vi "read error log.vi"() -> ()   [LabVIEW 2018]
panel:
  out "subarray 3":string[](array[string])
  out "subarray 2":string[](array[string])
  out "subarray":string[](array[string])
  out "Location Cluster out":T1
  in  "Tab Control":enum32{"Page 1", "Page 2", "Page 3"}(tab)
  out "Display":string[][](table)
  out "raw screen":string
  out "read":string
  out "text 2":string
  out "text":string
  out "all rows":string[][](array[string])
  out "Selection Position":cluster{i32, i32}={6, 2}
  in  "Stop":bool
  out "error out":errorcluster
  out "Source":string
  out "Code":string
  out "Timestamp":string
  in  "Numeric":i32
  # "is screen dimension check not working?? number of columns are counted in update display..."
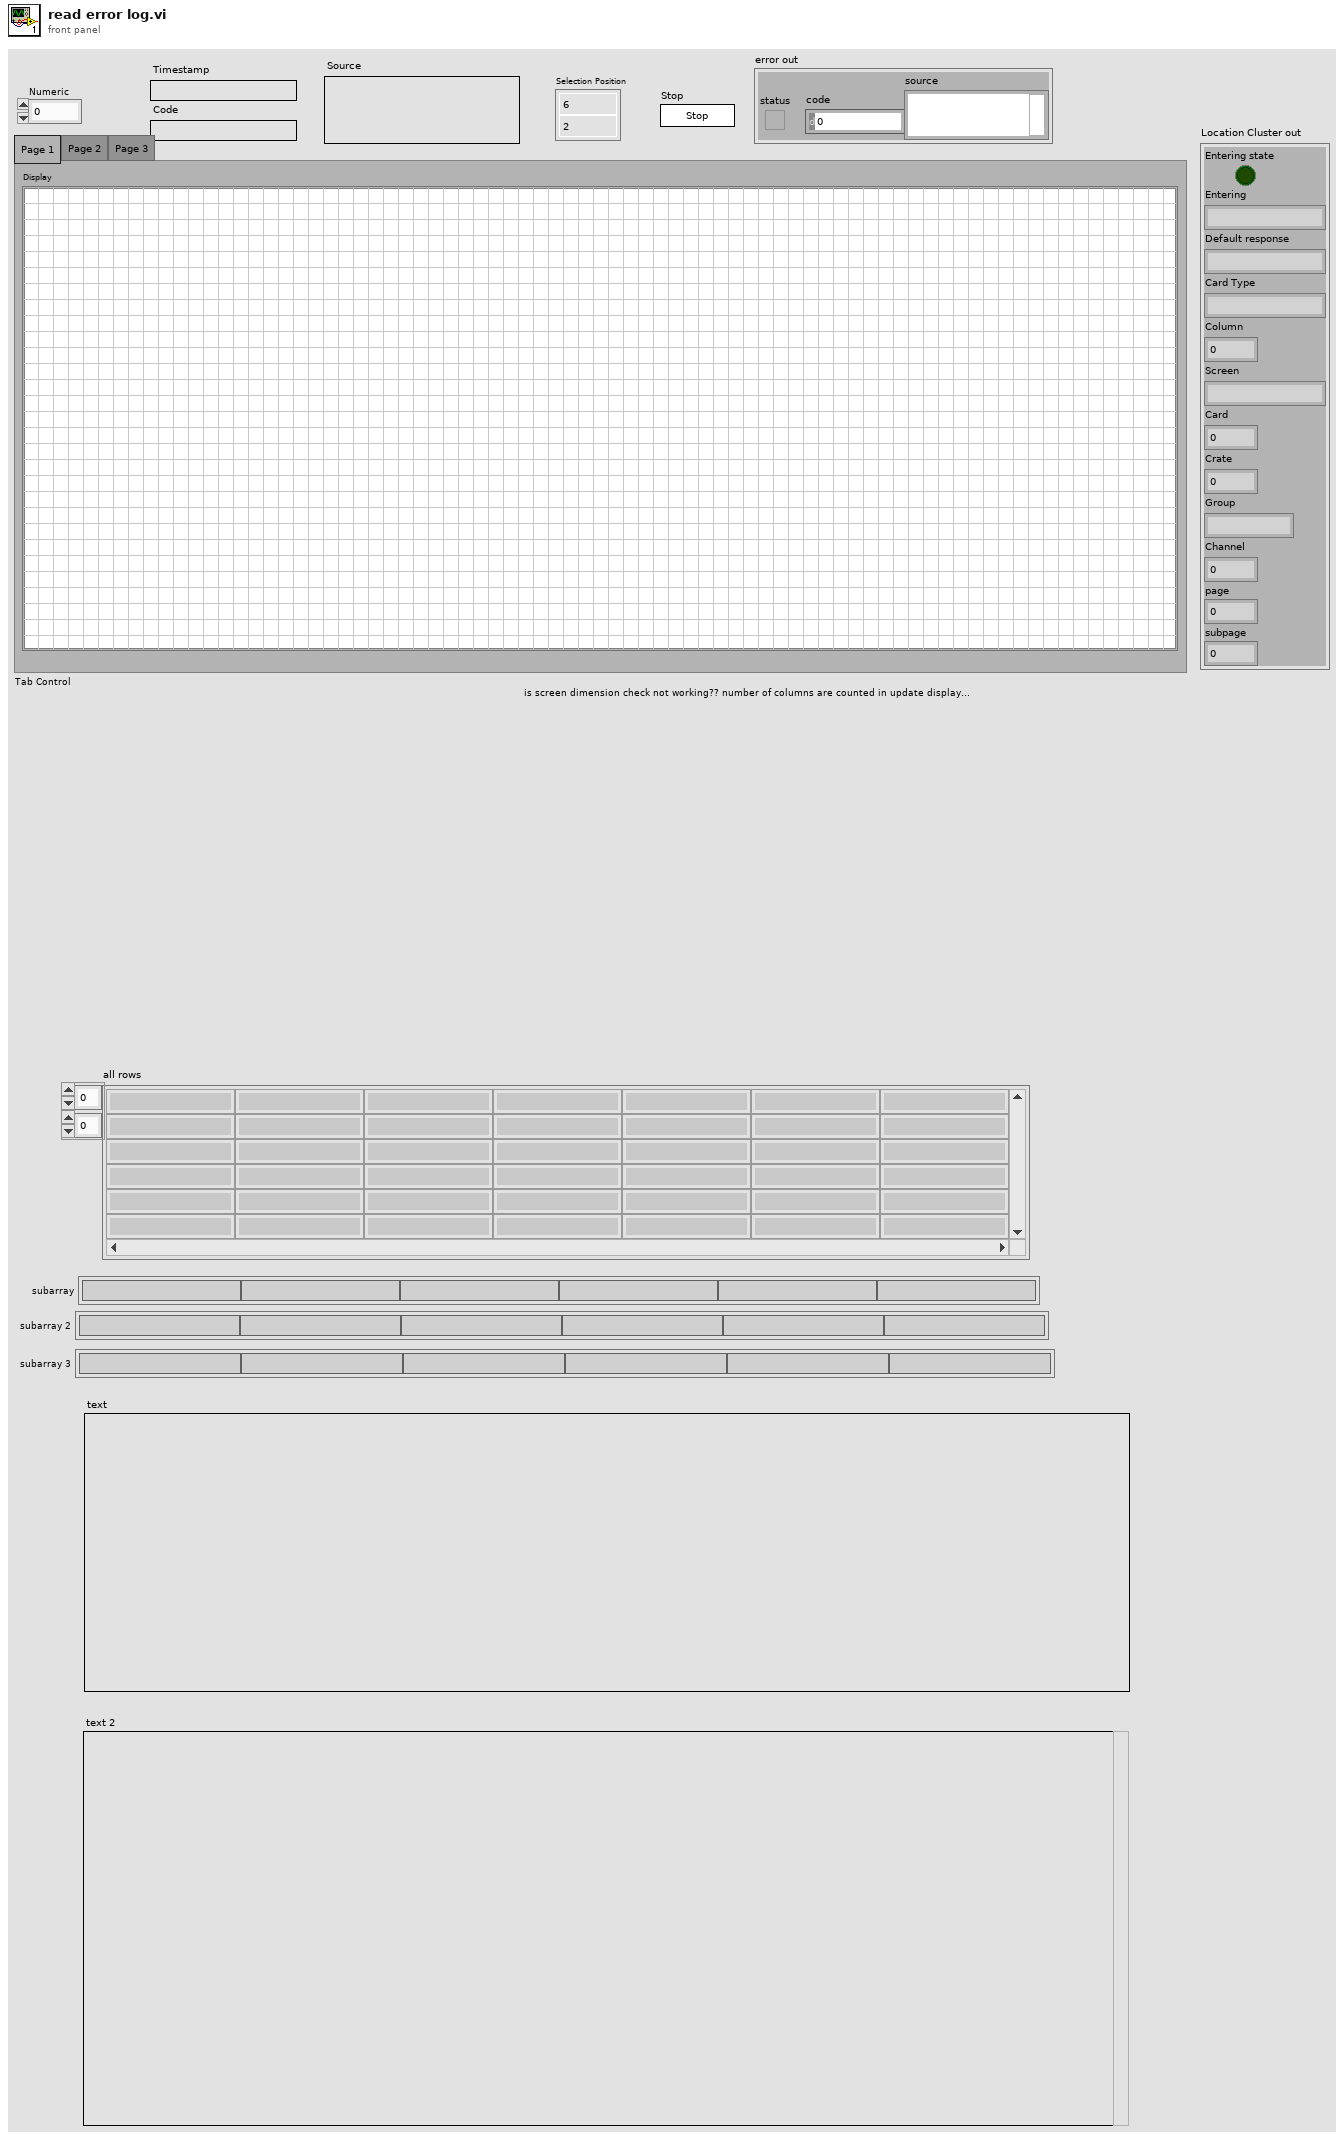
[diagram p1: front panel]
types:
  T1 = cluster{"Screen":string, "Crate":i32, "page":i32, "subpage":i32, "Entering state":bool, "Entering":string, "Default response":string, "Card":i32, "Channel":i32, "Card Type":string, "Column":i32, "Group":string}
  T2 = typedef "location cluster.ctl" = cluster{"Column":i32, "Card Type":string, "Channel":i32, "Card":i32, "Default response":string, "Entering":string, "Entering state":bool, "subpage":i32, "page":i32, "Crate":i32, "Screen":string, "Group":string, "Global HV Enable":bool}
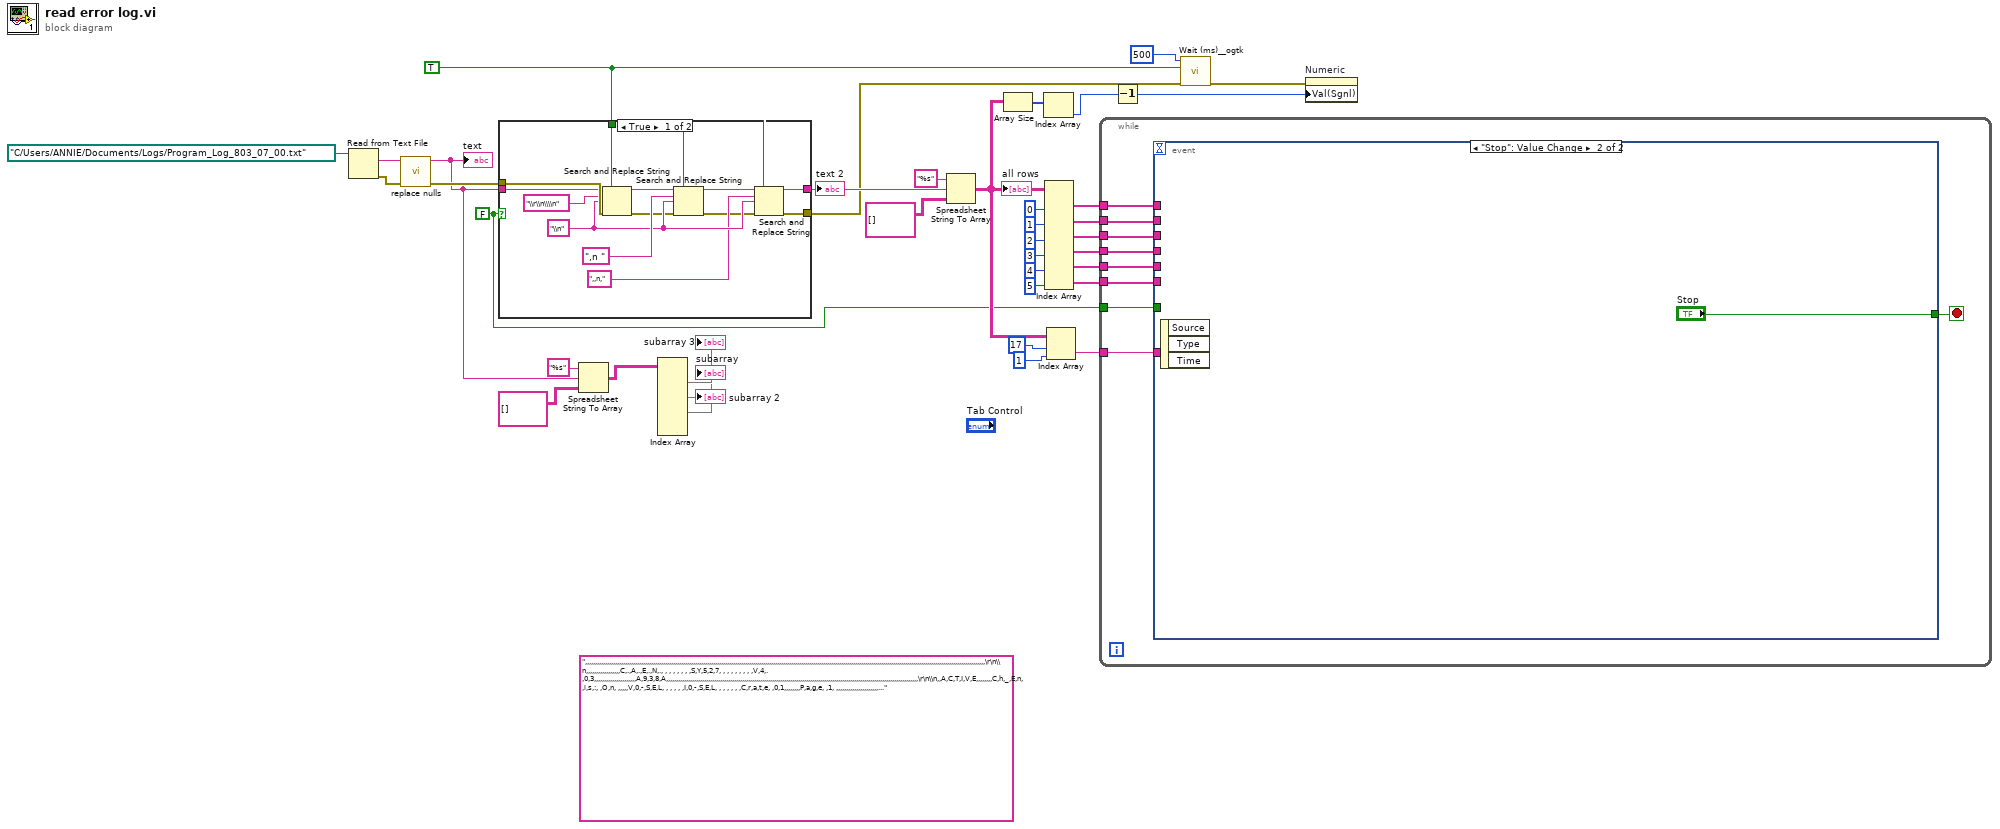
[diagram p0: block diagram]
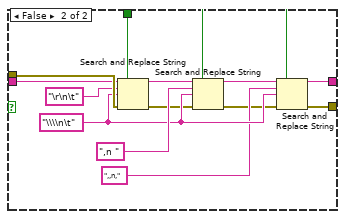
[diagram p2: hidden frame]
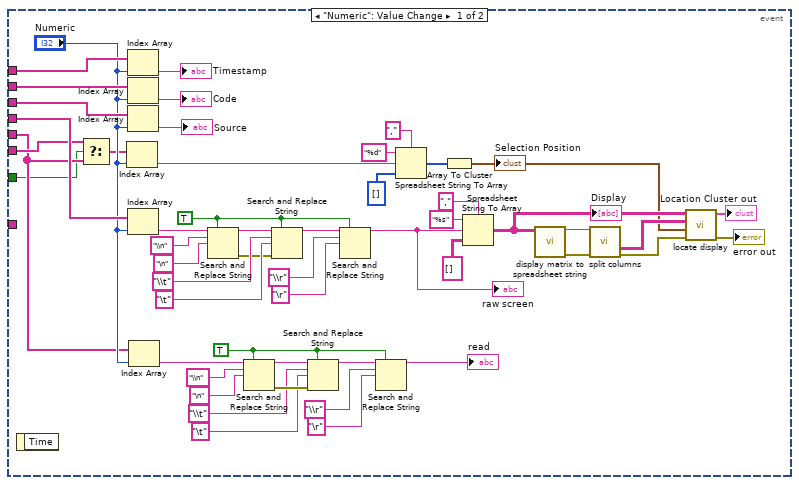
[diagram p3: hidden frame]
diagram:
  w1 = FALSE
  w17 = TRUE ("replace all? (F)")
  (unwired) ",,,,,,,,,,,,,,,,,,,,,,,,,,,,,,,,,,,,,,,,,,,,,,,,,,,,,,,,,,,,,,,,,,,,,,,,,,,,,,,,,,,,,,,,,,,,,,,,,,,,,,,,,,,,,,,,,,,,,,,,,,,,,,,,,,,,,,,,,,,,,,,,,,,,,,,,,,,,,,,,,,,,,,,,,,,,,,,,,,,,,,,,,,,,,,,,,,,,,,,,\r\n\\n,,,,,,,,,,,,,,,,,C,.,A,.,E,.,N,., , , , , , , ,S,Y,5,2,7, , , , , , , , ,V,4,.,0,3,,,,,,,,,,,,,,,,,,,,,A,9,3,8,A,,,,,,,,,,,,,,,,,,,,,,,,,,,,,,,,,,,,,,,,,,,,,,,,,,,,,,,,,,,,,,,,,,,,,,,,,,,,,,,,,,,,,,,,,,,,,,,,,,,,,,,,,,,,,,,,,,,,,,,,,,,,,,\r\n\\n,,A,C,T,I,V,E,,,,,,,,C,h,_,E,n, ,i,s,:, ,O,n, ,,,,,V,0,-,S,E,L, , , , , ,I,0,-,S,E,L, , , , , , ,C,r,a,t,e, ,0,1,,,,,,,,P,a,g,e, ,1, ,,,,,,,,,,,,,,,,,,,,,,,,,,,,,,,,,,,,,,,,,,,,,,,,,,,,,,,,,,,,,,,,,,,,,,,,,,,,,,,,,,,,,,,,,,,,,,,,,,,,,,,,,,,,,,,,,,,,,,,,,,,,\r\n\\n,,,,,,,,,,,,,,,,,,,,,,,,,,,,,,,,,,,,,,,,,,,,,,,,,,,,,,,,,,,,,,,,,,,,,,,,,,,,,,,,,,,,,,,,,,,,,,,,,,,,,,,,,,,,,,,,,,,,,,,,,,,,,,,,,,,,,,,,,,,,,,,,,,,,,,,,,,,,,,,,,,,,,,,,,,,,,,,,,,,,,,,,,,,,,,,,,,,,,,,,\r\n\\n, ,C,h,a,n,n,e,l, , , , , ,S,V,m,a,x, , ,R,u,p, , ,R,d,w,n, , ,T,r,i,p, ,T,r,i,p,E,x, ,P,r,O,n, ,P,r,O,f,f, ,P,o,n, , ,P,d,w,n, ,P,s,w,d, ,O,n,/,O,f,f, , ,C,h,#,,,,,,,,,,,,,,,,,,,,,,,,,,,,,,,,,,,,,,,,,,,,,,,,,,,,,,,,,,,,,,,,,,,,,,,,,,,,,,,,,,,,,,,,,,,,,,,,,,,,,,,,,,,,,,,,,,,,,,,,\r\n\\n, ,C,H,A,N,N,E,L,1,6, , , , ,2,0,0,0, , ,1,0,0, , ,1,0,0, , ,0,1,0,.,0, , , ,-,-, , , , ,0,1, , , ,0,1, , , ,O,f,f, , ,R,d,w,n, , , , , , , , , , , , , ,1,.,1,6,,,,,,,,,,,,,,,,,,,,,,,,,,,,,,,,,,,,,,,,,,,,,,,,,,,,,,,,,,,,,,,,,,,,,,,,,,,,,,,,,,,,,,,,,,,,,,,,,,,,,,,,,,,,,,,,,,,,,,,,\r\n\\n, ,C,H,A,N,N,E,L,1,7, , , , ,2,0,0,0, , ,1,0,0, , ,1,0,0, , ,0,1,0,.,0, , , ,-,-, , , , ,0,1, , , ,0,1, , , ,O,f,f, , ,R,d,w,n, , , , , , , , , , , , , ,1,.,1,7,,,,,,,,,,,,,,,,,,,,,,,,,,,,,,,,,,,,,,,,,,,,,,,,,,,,,,,,,,,,,,,,,,,,,,,,,,,,,,,,,,,,,,,,,,,,,,,,,,,,,,,,,,,,,,,,,,,,,,,,\r\n\\n, ,C,H,A,N,N,E,L,1,8, , , , ,2,0,0,0, , ,1,0,0, , ,1,0,0, , ,0,1,0,.,0, , , ,-,-, , , , ,0,1, , , ,0,1, , , ,O,f,f, , ,R,d,w,n, , , , , , , , , , , , , ,1,.,1,8,,,,,,,,,,,,,,,,,,,,,,,,,,,,,,,,,,,,,,,,,,,,,,,,,,,,,,,,,,,,,,,,,,,,,,,,,,,,,,,,,,,,,,,,,,,,,,,,,,,,,,,,,,,,,,,,,,,,,,,,\r\n\\n, ,C,H,A,N,N,E,L,1,9, , , , ,2,0,0,0, , ,1,0,0, , ,1,0,0, , ,0,1,0,.,0, , , ,-,-, , , , ,0,1, , , ,0,1, , , ,O,f,f, , ,R,d,w,n, , , , , , , , , , , , , ,1,.,1,9,,,,,,,,,,,,,,,,,,,,,,,,,,,,,,,,,,,,,,,,,,,,,,,,,,,,,,,,,,,,,,,,,,,,,,,,,,,,,,,,,,,,,,,,,,,,,,,,,,,,,,,,,,,,,,,,,,,,,,,,\r\n\\n, ,C,H,A,N,N,E,L,2,0, , , , ,2,0,0,0, , ,1,0,0, , ,1,0,0, , ,0,1,0,.,0, , , ,-,-, , , , ,0,1, , , ,0,1, , , ,O,f,f, , ,R,d,w,n, , , , , , , , , , , , , ,1,.,2,0,,,,,,,,,,,,,,,,,,,,,,,,,,,,,,,,,,,,,,,,,,,,,,,,,,,,,,,,,,,,,,,,,,,,,,,,,,,,,,,,,,,,,,,,,,,,,,,,,,,,,,,,,,,,,,,,,,,,,,,,\r\n\\n, ,C,H,A,N,N,E,L,2,1, , , , ,2,0,0,0, , ,1,0,0, , ,1,0,0, , ,0,1,0,.,0, , , ,-,-, , , , ,0,1, , , ,0,1, , , ,O,f,f, , ,R,d,w,n, , , , , , , , , , , , , ,1,.,2,1,,,,,,,,,,,,,,,,,,,,,,,,,,,,,,,,,,,,,,,,,,,,,,,,,,,,,,,,,,,,,,,,,,,,,,,,,,,,,,,,,,,,,,,,,,,,,,,,,,,,,,,,,,,,,,,,,,,,,,,,\r\n\\n, ,C,H,A,N,N,E,L,2,2, , , , ,2,0,0,0, , ,1,0,0, , ,1,0,0, , ,0,1,0,.,0, , , ,-,-, , , , ,0,1, , , ,0,1, , , ,O,f,f, , ,R,d,w,n, , , , , , , , , , , , , ,1,.,2,2,,,,,,,,,,,,,,,,,,,,,,,,,,,,,,,,,,,,,,,,,,,,,,,,,,,,,,,,,,,,,,,,,,,,,,,,,,,,,,,,,,,,,,,,,,,,,,,,,,,,,,,,,,,,,,,,,,,,,,,,\r\n\\n, ,C,H,A,N,N,E,L,2,3, , , , ,2,0,0,0, , ,1,0,0, , ,1,0,0, , ,0,1,0,.,0, , , ,-,-, , , , ,0,1, , , ,0,1, , , ,O,f,f, , ,R,d,w,n, , , , , , , , , , , , , ,1,.,2,3,,,,,,,,,,,,,,,,,,,,,,,,,,,,,,,,,,,,,,,,,,,,,,,,,,,,,,,,,,,,,,,,,,,,,,,,,,,,,,,,,,,,,,,,,,,,,,,,,,,,,,,,,,,,,,,,,,,,,,,,\r\n\\n, ,C,H,A,N,N,E,L,2,4, , , , ,2,0,0,0, , ,1,0,0, , ,1,0,0, , ,0,1,0,.,0, , , ,-,-, , , , ,0,1, , , ,0,1, , , ,O,f,f, , ,R,d,w,n, , , , , , , , , , , , , ,1,.,2,4,,,,,,,,,,,,,,,,,,,,,,,,,,,,,,,,,,,,,,,,,,,,,,,,,,,,,,,,,,,,,,,,,,,,,,,,,,,,,,,,,,,,,,,,,,,,,,,,,,,,,,,,,,,,,,,,,,,,,,,,\r\n\\n, ,C,H,A,N,N,E,L,0,0, , , , ,2,0,0,0, , ,1,0,0, , ,1,0,0, , ,0,1,0,.,0, , , ,-,-, , , , ,0,1, , , ,0,1, , , ,O,f,f, , ,R,d,w,n, , , , , , , , , , , , , ,2,.,0,0,,,,,,,,,,,,,,,,,,,,,,,,,,,,,,,,,,,,,,,,,,,,,,,,,,,,,,,,,,,,,,,,,,,,,,,,,,,,,,,,,,,,,,,,,,,,,,,,,,,,,,,,,,,,,,,,,,,,,,,,\r\n\\n, ,C,H,A,N,N,E,L,0,1, , , , ,2,0,0,0, , ,1,0,0, , ,1,0,0, , ,0,1,0,.,0, , , ,-,-, , , , ,0,1, , , ,0,1, , , ,O,f,f, , ,R,d,w,n, , , , , , , , , , , , , ,2,.,0,1,,,,,,,,,,,,,,,,,,,,,,,,,,,,,,,,,,,,,,,,,,,,,,,,,,,,,,,,,,,,,,,,,,,,,,,,,,,,,,,,,,,,,,,,,,,,,,,,,,,,,,,,,,,,,,,,,,,,,,,,\r\n\\n, ,C,H,A,N,N,E,L,0,2, , , , ,2,0,0,0, , ,1,0,0, , ,1,0,0, , ,0,1,0,.,0, , , ,-,-, , , , ,0,1, , , ,0,1, , , ,O,f,f, , ,R,d,w,n, , , , , , , , , , , , , ,2,.,0,2,,,,,,,,,,,,,,,,,,,,,,,,,,,,,,,,,,,,,,,,,,,,,,,,,,,,,,,,,,,,,,,,,,,,,,,,,,,,,,,,,,,,,,,,,,,,,,,,,,,,,,,,,,,,,,,,,,,,,,,,\r\n\\n, ,C,H,A,N,N,E,L,0,3, , , , ,2,0,0,0, , ,1,0,0, , ,1,0,0, , ,0,1,0,.,0, , , ,-,-, , , , ,0,1, , , ,0,1, , , ,O,f,f, , ,R,d,w,n, , , , , , , , , , , , , ,2,.,0,3,,,,,,,,,,,,,,,,,,,,,,,,,,,,,,,,,,,,,,,,,,,,,,,,,,,,,,,,,,,,,,,,,,,,,,,,,,,,,,,,,,,,,,,,,,,,,,,,,,,,,,,,,,,,,,,,,,,,,,,,\r\n\\n, ,C,H,A,N,N,E,L,0,4, , , , ,2,0,0,0, , ,1,0,0, , ,1,0,0, , ,0,1,0,.,0, , , ,-,-, , , , ,0,1, , , ,0,1, , , ,O,f,f, , ,R,d,w,n, , , , , , , , , , , , , ,2,.,0,4,,,,,,,,,,,,,,,,,,,,,,,,,,,,,,,,,,,,,,,,,,,,,,,,,,,,,,,,,,,,,,,,,,,,,,,,,,,,,,,,,,,,,,,,,,,,,,,,,,,,,,,,,,,,,,,,,,,,,,,,\r\n\\n, ,C,H,A,N,N,E,L,0,5, , , , ,1,8,0,0, , ,1,0,0, , ,1,0,0, , ,0,1,0,.,0, , , ,-,-, , , , ,0,1, , , ,0,1, , , ,O,f,f, , ,R,d,w,n, , , , , , , , , , , , , ,2,.,0,5,,,,,,,,,,,,,,,,,,,,,,,,,,,,,,,,,,,,,,,,,,,,,,,,,,,,,,,,,,,,,,,,,,,,,,,,,,,,,,,,,,,,,,,,,,,,,,,,,,,,,,,,,,,,,,,,,,,,,,,,\r\n\\n, ,C,H,A,N,N,E,L,0,6, , , , ,1,8,0,0, , ,1,0,0, , ,1,0,0, , ,0,1,0,.,0, , , ,-,-, , , , ,0,1, , , ,0,1, , , ,O,f,f, , ,R,d,w,n, , , , , , , , , , , , , ,2,.,0,6,,,,,,,,,,,,,,,,,,,,,,,,,,,,,,,,,,,,,,,,,,,,,,,,,,,,,,,,,,,,,,,,,,,,,,,,,,,,,,,,,,,,,,,,,,,,,,,,,,,,,,,,,,,,,,,,,,,,,,,,\r\n\\n,,,,,,,,,,,,,,,,,,,,,,,,,,,,,,,,,,,,,,,,,,,,,,,,,,,,,,,,,,,,,,,,,,,,,,,,,,,,,,,,,,,,,,,,,,,,,,,,,,,,,,,,,,,,,,,,,,,,,,,,,,,,,,,,,,,,,,,,,,,,,,,,,,,,,,,,,,,,,,,,,,,,,,,,,,,,,,,,,,,,,,,,,,,,,,,,,,,,,,,,\r\n\\n,,,,,,,,,,,,,,,,,,,,,,,,,,,,,,,,,,,,,,,,,,,,,,,,,,,,,,,,,,,,,,,,,,,,,,,,,,,,,,,,,,,,,,,,,,,,,,,,,,,,,,,,,,,,,,,,,,,,,,,,,,,,,,,,,,,,,,,,,,,,,,,,,,,,,,,,,,,,,,,,,,,,,,,,,,,,,,,,,,,,,,,,,,,,,,,,,,,,,,,,\r\n\\n,,,,,,,,,,,,,,,,,,,,,,,,,,,,,,,,,,,,,,,,,,,,,,,,,,,,,,,,,,,,,,,,,,,,,,,,,,,,,,,,,,,,,,,,,,,,,,,,,,,,,,,,,,,,,,,,,,,,,,,,,,,,,,,,,,,,,,,,,,,,,,,,,,,,,,,,,,,,,,,,,,,,,,,,,,,,,,,,,,,,,,,,,,,,,,,,,,,,,,,,\r\n\\n, ,Q,u,i,t, ,E,d,i,t, ,C,h,a,n,g,e, ,A,d,d, ,I,n,s,e,r,t, ,R,e,p,l,a,c,e, ,D,e,l,e,t,e, ,U,p,d,a,t,e, ,N,e,x,t, ,P,r,e,v, ,M,o,r,e, ,S,w,i,t,c,h,,,,,,,,,,,,,,,,,,,,,,,,,,,,,,,,,,,,,,,,,,,,,,,,,,,,,,,,,,,,,,,,,,,,,,,,,,,,,,,,,,,,,,,,,,,,,,,,,,,,,,,,,,,,,,,,,,,,,,,,,,,,,,,,\r\n\\n,,,,,,,,,,,,,,,,,,,,,,,,,,,,,,,,,,,,,,,,,,,,,,,,,,,,,,,,,,,,,,,,,,,,,,,,,,,,,,,,,,,,,,,,,,,,,,,,,,,,,,,,,,,,,,,,,,,,,,,,,,,,,,,,,,,,,,,,,,,,,,,,,,,,,,,,,,,,,,,,,,,,,,,,,,,,,,,,,,,,,,,,,,,,,,,,,,,,,,,,\r\n\\n,,,,,,,,,,,,,,,,,,,,,,,,,,,,,,,,,,,,,,,,,,,,,,,,,,,,,,,,,,,,,,,,,,,,,,,,,,,,,,,,,,,,,,,,,,,,,,,,,,,,,,,,,,,,,,,,,,,,,,,,,,,,,,,,,,,,,,,,,,,,,,,,,,,,,,,,,,,,,,,,,,,,,,,,,,,,,,,,,,,,,,,,,,,,,,,,,,,,,,,,\r\n\\n,,,,,,,,,,,,,,,,,,,,,,,,,,,,,,,,,,,,,,,,,,,,,,,,,,,,,,,,,,,,,,,,,,,,,,,,,,,,,,,,,,,,,,,,,,,,,,,,,,,,,,,,,,,,,,,,,,,,,,,,,,,,,,,,,,,,,,,,,,,,,,,,,,,,,,,,,,,,,,,,,,,,,,,,,,,,,,,,,,,,,,,,,,,,,,,,,,,,,,,,\r\n\\n,,,,,,,,,,,,,,,,,,,,,,,,,,,,,,,,,,,,,,,,,,,,,,,,,,,,,,,,,,,,,,,,,,,,,,,,,,,,,,,,,,,,,,,,,,,,,,,,,,,,,,,,,,,,,,,,,,,,,,,,,,,,,,,,,,,,,,,,,,,,,,,,,,,,,,,,,,,,,,,,,,,,,,,,,,,,,,,,,,,,,,,,,,,,,,,,,,,,,,,,\r\n\\n,,,,,,,,,,,,,,,,,,,,,,,,,,,,,,,,,,,,,,,,,,,,,,,,,,,,,,,,,,,,,,,,,,,,,,,,,,,,,,,,,,,,,,,,,,,,,,,,,,,,,,,,,,,,,,,,,,,,,,,,,,,,,,,,,,,,,,,,,,,,,,,,,,,,,,,,,,,,,,,,,,,,,,,,,,,,,,,,,,,,,,,,,,,,,,,,,,,,,,,,\r\n\\n,,,,,,,,,,,,,,,,,,,,,,,,,,,,,,,,,,,,,,,,,,,,,,,,,,,,,,,,,,,,,,,,,,,,,,,,,,,,,,,,,,,,,,,,,,,,,,,,,,,,,,,,,,,,,,,,,,,,,,,,,,,,,,,,,,,,,,,,,,,,,,,,,,,,,,,,,,,,,,,,,,,,,,,,,,,,,,,,,,,,,,,,,,,,,,,,,,,,,,,,\r\n\\n,,,,,,,,,,,,,,,,,,,,,,,,,,,,,,,,,,,,,,,,,,,,,,,,,,,,,,,,,,,,,,,,,,,,,,,,,,,,,,,,,,,,,,,,,,,,,,,,,,,,,,,,,,,,,,,,,,,,,,,,,,,,,,,,,,,,,,,,,,,,,,,,,,,,,,,,,,,,,,,,,,,,,,,,,,,,,,,,,,,,,,,,,,,,,,,,,,,,,,,,\r\n\\n,,,,,,,,,,,,,,,,,,,,,,,,,,,,,,,,,,,,,,,,,,,,,,,,,,,,,,,,,,,,,,,,,,,,,,,,,,,,,,,,,,,,,,,,,,,,,,,,,,,,,,,,,,,,,,,,,,,,,,,,,,,,,,,,,,,,,,,,,,,,,,,,,,,,,,,,,,,,,,,,,,,,,,,,,,,,,,,,,,,,,,,,,,,,,,,,,,,,,,,,\r\n\\n,,,,,,,,,,,,,,,,,,,,,,,,,,,,,,,,,,,,,,,,,,,,,,,,,,,,,,,,,,,,,,,,,,,,,,,,,,,,,,,,,,,,,,,,,,,,,,,,,,,,,,,,,,,,,,,,,,,,,,,,,,,,,,,,,,,,,,,,,,,,,,,,,,,,,,,,,,,,,,,,,,,,,,,,,,,,,,,,,,,,,,,,,,,,,,,,,,,,,,,,\r\n\\n,,,,,,,,,,,,,,,,,,,,,,,,,,,,,,,,,,,,,,,,,,,,,,,,,,,,,,,,,,,,,,,,,,,,,,,,,,,,,,,,,,,,,,,,,,,,,,,,,,,,,,,,,,,,,,,,,,,,,,,,,,,,,,,,,,,,,,,,,,,,,,,,,,,,,,,,,,,,,,,,,,,,,,,,,,,,,,,,,,,,,,,,,,,,,,,,,,,,,,,,\r\n\\n,,,,,,,,,,,,,,,,,,,,,,,,,,,,,,,,,,,,,,,,,,,,,,,,,,,,,,,,,,,,,,,,,,,,,,,,,,,,,,,,,,,,,,,,,,,,,,,,,,,,,,,,,,,,,,,,,,,,,,,,,,,,,,,,,,,,,,,,,,,,,,,,,,,,,,,,,,,,,,,,,,,,,,,,,,,,,,,,,,,,,,,,,,,,,,,,,,,,,,,,\r\n\\n,,,,,,,,,,,,,,,,,,,,,,,,,,,,,,,,,,,,,,,,,,,,,,,,,,,,,,,,,,,,,,,,,,,,,,,,,,,,,,,,,,,,,,,,,,,,,,,,,,,,,,,,,,,,,,,,,,,,,,,,,,,,,,,,,,,,,,,,,,,,,,,,,,,,,,,,,,,,,,,,,,,,,,,,,,,,,,,,,,,,,,,,,,,,,,,,,,,,,,,,\r\n\\n,,,,,,,,,,,,,,,,,,,,,,,,,,,,,,,,,,,,,,,,,,,,,,,,,,,,,,,,,,,,,,,,,,,,,,,,,,,,,,,,,,,,,,,,,,,,,,,,,,,,,,,,,,,,,,,,,,,,,,,,,,,,,,,,,,,,,,,,,,,,,,,,,,,,,,,,,,,,,,,,,,,,,,,,,,,,,,,,,,,,,,,,,,,,,,,,,,,,,,,,\r\n\\n,,,,,,,,,,,,,,,,,,,,,,,,,,,,,,,,,,,,,,,,,,,,,,,,,,,,,,,,,,,,,,,,,,,,,,,,,,,,,,,,,,,,,,,,,,,,,,,,,,,,,,,,,,,,,,,,,,,,,,,,,,,,,,,,,,,,,,,,,,,,,,,,,,,,,,,,,,,,,,,,,,,,,,,,,,,,,,,,,,,,,,,,,,,,,,,,,,,,,,,,\r\n\\n,,,,,,,,,,,,,,,,,,,,,,,,,,,,,,,,,,,,,,,,,,,,,,,,,,,,,,,,,,,,,,,,,,,,,,,,,,,,,,,,,,,,,,,,,,,,,,,,,,,,,,,,,,,,,,,,,,,,,,,,,,,,,,,,,,,,,,,,,,,,,,,,,,,,,,,,,,,,,,,,,,,,,,,,,,,,,,,,,,,,,,,,,,,,,,,,,,,,,,,,\r\n\\n,,,,,,,,,,,,,,,,,,,,,,,,,,,,,,,,,,,,,,,,,,,,,,,,,,,,,,,,,,,,,,,,,,,,,,,,,,,,,,,,,,,,,,,,,,,,,,,,,,,,,,,,,,,,,,,,,,,,,,,,,,,,,,,,,,,,,,,,,,,,,,,,,,,,,,,,,,,,,,,,,,,,,,,,,,,,,,,,,,,,,,,,,,,,,,,,,,,,,,,,\r\n\\n" ("format string")
  n1 = Read from Text File(file (use dialog)=path "C:/Users/ANNIE/Documents/Logs/Program_Log_803_07_00.txt" ("file path (dialog if empty)")) -> (text=w15:string, error out=w13:errorcluster)  [unwired: 3 in, 2 out]
  n2 = call "replace nulls.vi"("error in (no error)"=w13, "read buffer"=w15) -> ("error out"=w14:errorcluster, "result string"=w6:string)  [unwired: 8 in]
  "text" <- w6
  n3 = case shown="True" w1 {
    tunnel: [w51 w64] -> w23
    tunnel: w17 -> [w50 w63]
    tunnel: [w49 w62] -> w16
    tunnel: w14 -> [w48 w61]
    tunnel: w6 -> [w47 w60]
    frame True {
      w42 = "\\n" ("format string")
      n4 = Search and Replace String(replace all?=w50, input string=w47, search string="\\r\\n\\\\n" ("format string"), replace string=w42, error in=w48) -> (result string=w45:string, error out=w40:errorcluster)  [unwired: 3 in, 2 out]
      n5 = Search and Replace String(replace all?=w50, input string=w45, search string=",n " ("format string"), replace string=w42, error in=w40) -> (result string=w43:string, error out=w39:errorcluster)  [unwired: 3 in, 2 out]
      n6 = Search and Replace String(replace all?=w50, input string=w43, search string=",,n," ("format string"), replace string=w42, error in=w39) -> (result string=w51:string, error out=w49:errorcluster)  [unwired: 3 in, 2 out]
    }
    frame False {
      w55 = "\\\\n\t" ("format string")
      n7 = Search and Replace String(replace all?=w63, input string=w60, search string="\r\n\t" ("format string"), replace string=w55, error in=w61) -> (result string=w58:string, error out=w53:errorcluster)  [unwired: 3 in, 2 out]
      n8 = Search and Replace String(replace all?=w63, input string=w58, search string=",n " ("format string"), replace string=w55, error in=w53) -> (result string=w56:string, error out=w52:errorcluster)  [unwired: 3 in, 2 out]
      n9 = Search and Replace String(replace all?=w63, input string=w56, search string=",,n," ("format string"), replace string=w55, error in=w52) -> (result string=w64:string, error out=w62:errorcluster)  [unwired: 3 in, 2 out]
    }
  }
  "text 2" <- w23
  n10 = Spreadsheet String To Array(format string="%s", spreadsheet string=w6, array type (2D Dbl)=string[][] [] ("all rows")) -> (array=w5:string[][])  [unwired: 1 in]
  n11 = Index Array(array=w5) -> (element #1=→"subarray":string[], element #2=→"subarray 2":string[], element #3=→"subarray 3":string[])  [unwired: 8 in, 1 out]
  n12 = Spreadsheet String To Array(format string="%s", spreadsheet string=w23, array type (2D Dbl)=string[][] [] ("all rows")) -> (array=w12:string[][])  [unwired: 1 in]
  "all rows" <- w12
  n13 = Array Size(array=w12) -> (size(s)=w22:i32[])
  n14 = Index Array(array=w22) -> (element=w21:i32)  [unwired: 1 in]
  n15 = Index Array(array=w12, index (col) #1=0 ("index (row)"), index (col) #2=1 ("index (row)"), index (col) #3=2 ("index (row)"), index (col) #4=3 ("index (row)"), index (col) #5=4 ("index (row)"), index (col) #6=5 ("index (row)")) -> (element #1=w38:string[], element #2=w37:string[], element #3=w36:string[], element #4=w35:string[], element #5=w29:string[], element #6=w18:string[])  [unwired: 6 in]
  n16 = Index Array(array=w12, index (row)=17, index (col)=1 ("index (row)")) -> (element=w9:string)
  n17 = while {
    tunnel: w38 -> [w73]
    tunnel: w37 -> [w72]
    tunnel: w36 -> [w71]
    tunnel: w35 -> [w70]
    tunnel: w29 -> [w68]
    tunnel: w18 -> [w67]
    tunnel: w9 -> [w66]
    tunnel: w1 -> [w65]
    stop <- w69 stop-if-true
    n18 = event shown="[1] \"Stop\": Value Change" {
      selector: _ -> [_ _]
      dyn-events: _ -> [_ _]
      timeout: _ -> [_ _]
      tunnel: w73 -> [w125 _]
      tunnel: w72 -> [w124 _]
      tunnel: w71 -> [w123 _]
      tunnel: w70 -> [w81 _]
      tunnel: [_ "Stop"] -> w69
      tunnel: w68 -> [w76 _]
      tunnel: w67 -> [w77 _]
      tunnel: w66 -> [_ _]
      tunnel: w65 -> [w74 _]
      event "Numeric": Value Change {
        w90 = TRUE ("replace all? (F)")
        w96 = TRUE ("replace all? (F)")
        n19 = event-data() -> ()  [unwired: 1 in, 1 out]
        n20 = Select(t=w77, s=w74, f=w76) -> (s? t:f=w75:string[])
        n21 = Index Array(array=w75, index="Numeric") -> (element=w107:string)
        n22 = Index Array(array=w125, index="Numeric") -> (element=→"Timestamp":string)
        n23 = Index Array(array=w124, index="Numeric") -> (element=→"Code":string)
        n24 = Index Array(array=w123, index="Numeric") -> (element=→"Source":string)
        n25 = Index Array(array=w81, index="Numeric") -> (element=w78:string)
        n26 = Index Array(array=w76, index="Numeric") -> (element=w82:string)
        n27 = Search and Replace String(replace all?=w96, input string=w78, search string="\\n" ("format string"), replace string="\n" ("format string")) -> (result string=w100:string, error out=w99:errorcluster)  [unwired: 4 in, 2 out]
        n28 = Search and Replace String(replace all?=w90, input string=w82, search string="\\n" ("format string"), replace string="\n" ("format string")) -> (result string=w87:string, error out=w88:errorcluster)  [unwired: 4 in, 2 out]
        n29 = Search and Replace String(replace all?=w96, input string=w100, search string="\\t" ("input string"), replace string="\t" ("input string"), error in=w99) -> (result string=w98:string)  [unwired: 3 in, 3 out]
        n30 = Search and Replace String(replace all?=w90, input string=w87, search string="\\t" ("input string"), replace string="\t" ("input string"), error in=w88) -> (result string=w89:string)  [unwired: 3 in, 3 out]
        n31 = Search and Replace String(replace all?=w96, input string=w98, search string="\\r" ("format string"), replace string="\r" ("format string")) -> (result string=w97:string)  [unwired: 4 in, 3 out]
        "raw screen" <- w97
        n32 = Search and Replace String(replace all?=w90, input string=w89, search string="\\r" ("format string"), replace string="\r" ("format string")) -> (result string=→"read":string)  [unwired: 4 in, 3 out]
        n33 = Spreadsheet String To Array(delimiter (Tab)=",", format string="%d", spreadsheet string=w107, array type (2D Dbl)=i32[] [] ("Display")) -> (array=w106:i32[])
        n34 = Array To Cluster(array=w106) -> (cluster=w105:cluster{"Display[0]":i32, "Display[1]":i32})
        "Selection Position" <- w105
        n35 = Spreadsheet String To Array(delimiter (Tab)=",", format string="%s", spreadsheet string=w97, array type (2D Dbl)=string[][] [] ("Display")) -> (array=w117:string[][])
        "Display" <- w117
        n36 = call "display matrix to spreadsheet string.vi"("Display"=w117) -> ("error out"=w113:errorcluster, "spreadsheet string"=w116:string)  [unwired: 7 in, 2 out]
        n37 = call "split columns.vi"("Display string"=w116, "error in"=w113) -> ("Array"=w115:string[][], "error out"=w114:errorcluster)  [unwired: 9 in, 3 out]
        n38 = call "locate display.vi"("error in"=w114, "Selection Position"=w105, "Display array"=w115, "Display"=w117) -> ("error out"=→"error out":errorcluster, "Location Cluster out"=→"Location Cluster out":T2)  [unwired: 6 in]
      }
      event "Stop": Value Change {
        n39 = event-data() -> ()  [unwired: 1 in, 3 out]
      }
    }
  }
  n40 = Decrement(x=w21) -> (x-1=w20:i32)
  n41 = call <userlib>:"Wait (ms)__ogtk.vi"("error in (no error)"=w16, "Wait on Error (FALSE)"=w17, "milliseconds to wait"=500 ("Value (Signaling)")) -> ("error out"=w28:errorcluster)  [unwired: 7 in, 1 out]
  n42 = property on="Numeric" class="DigNum (strict)"(error in=w28, "Val(Sgnl)"=w20) -> ()  [unwired: 1 in, 2 out]
